vi "send_email.vi"(9 "email list":string[](array[string])=["kalicy@cua.edu", "stara@jlab.org", "bgreg@jlab.org", "svarrigo@jlab.org", "andrewl@jlab.org", "tlemon@jlab.org"], 10 "log-path":path, 11 "max-only path":path) -> ()   [LabVIEW 2024]
uses:
  <vilib>/Utility/error.llb/Trim Whitespace One-Sided.vi
  <vilib>/smtpClient/Set Message Text.vi
  <vilib>/smtpClient/LabVIEWSMTPClient.lvlib
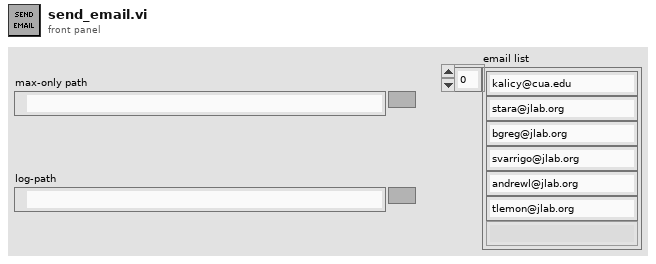
[diagram p1: front panel]
types:
  T1 = typedef "LabVIEWSMTPClient.lvlib/SmtpClientHandle.ctl" = refnum<k1>
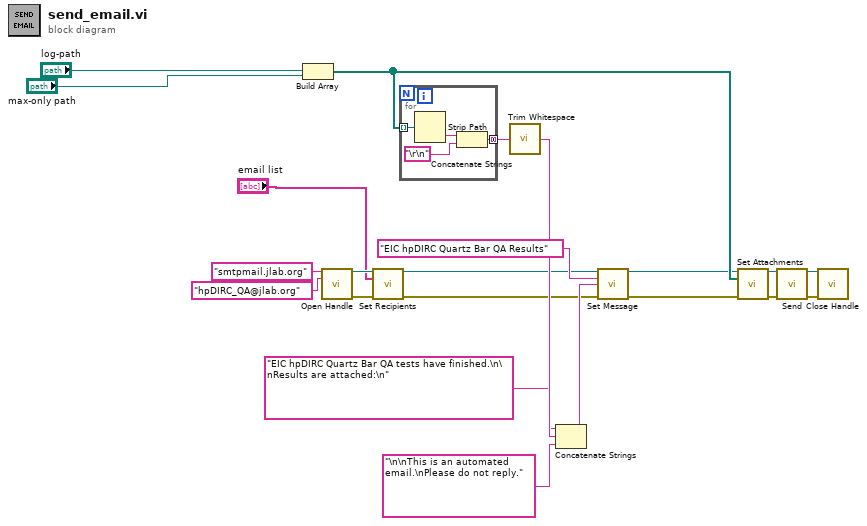
[diagram p0: block diagram]
diagram:
  n1 = Build Array("log-path", "max-only path") -> (w17:path[])
  n2 = call <vilib>:"Open Handle.vi"("server address"="smtpmail.jlab.org", "from"="hpDIRC_QA@jlab.org") -> ("handle out"=w4:T1, "error out"=w5:errorcluster)  [unwired: 12 in]
  n3 = call <vilib>:"Set Recipients.vi"("handle in"=w4, "to"="email list", "error in (no error)"=w5) -> ("handle out"=w6:T1, "error out"=w7:errorcluster)  [unwired: 11 in]
  n4 = for {
    tunnel: w17 -> [w26] mode=indexing
    tunnel: [w24] -> w18 mode=concatenating
    n5 = Strip Path(path=w26) -> (name=w25:string)  [unwired: 1 out]
    n6 = Concatenate Strings(w25, "\r\n") -> (w24:string)
  }
  n7 = call <vilib>:"Trim Whitespace.vi"("string"=w18) -> ("trimmed string"=w21:string)  [unwired: 1 in]
  n8 = Concatenate Strings("EIC hpDIRC Quartz Bar QA tests have finished.\n\nResults are attached:\n" ("plain text message"), w21, "\n\nThis is an automated email.\nPlease do not reply." ("string")) -> (w20:string)
  n9 = call-poly <vilib>:"Set Message.vi"("handle in"=w6, "subject"="EIC hpDIRC Quartz Bar QA Results", "plain text message"=w20, "error in (no error)"=w7) -> ("handle out"=w10:T1, "error out"=w11:errorcluster)  [unwired: 10 in]
  n10 = call <vilib>:"Set Attachments.vi"("handle in"=w10, "attachments"=w17, "error in (no error)"=w11) -> ("handle out"=w12:T1, "error out"=w13:errorcluster)  [unwired: 11 in]
  n11 = call <vilib>:"Send.vi"("handle in"=w12, "error in (no error)"=w13) -> ("handle out"=w14:T1, "error out"=w15:errorcluster)  [unwired: 11 in, 1 out]
  n12 = call <vilib>:"Close Handle.vi"("handle in"=w14, "error in (no error)"=w15) -> ()  [unwired: 12 in, 2 out]
